vi "ActionVIOnLoad.vi"(8 "error in":errorcluster, 11 "Device Item Ref in":T1 format="%.0x") -> (0 "error out":errorcluster, 3 "Device Item Ref out":T1 format="%.0x")   [LabVIEW 2020, in "AIM MIL-STD-1553 System Explorer.lvlib" / "Implementation.lvlib"]
uses:
  Implementation.lvlib
  <vilib>/NI VeriStand/Custom Device API/Custom Device API.lvlib
  NationalInstruments.VeriStand.SystemDefinitionAPI
  Scripting/AIM MIL-STD-1553 Scripting.lvlib
  <vilib>/NI VeriStand/Custom Device API/Custom Device Item Ref.ctl
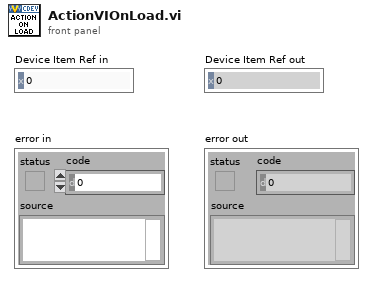
[diagram p1: front panel]
types:
  T1 = typedef "Custom Device API.lvlib/Custom Device Item Ref.ctl" = u64
  T2 = typedef "Custom Device API.lvlib/Custom Device Item Info.ctl" = cluster{"Name":string, "Is Channel":bool, "GUID":string, "Is Waveform":bool}
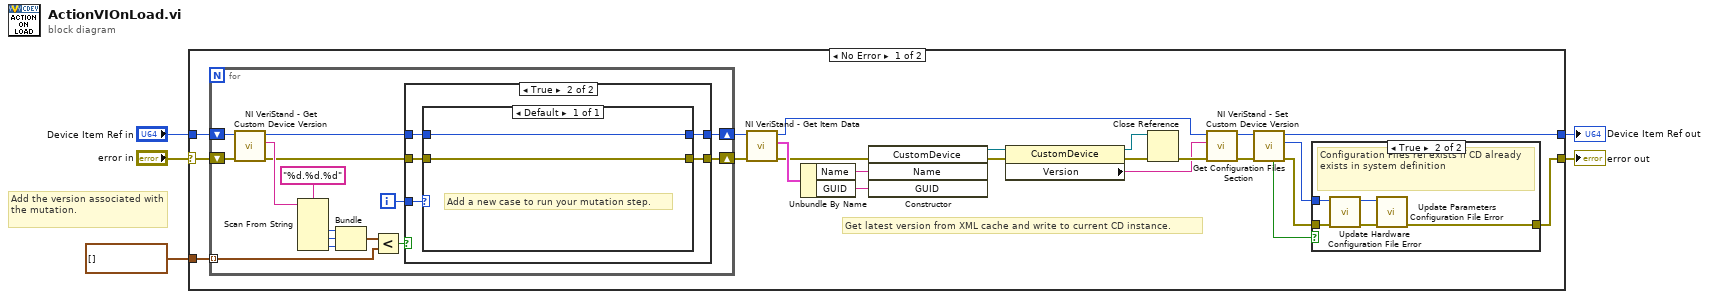
[diagram p0: block diagram]
diagram:
  # "Add the version associated with the mutation."
  n1 = case shown="No Error" "error in" {
    selector: "error in" -> [w28 w60]
    tunnel: [w8 w60] -> w3
    tunnel: "Device Item Ref in" -> [w27 w59]
    tunnel: [w7 w59] -> w2
    tunnel: cluster{i32, i32, i32}[] [] -> [w26 _]
    frame No Error {
      # "Get latest version from XML cache and write to current CD instance."
      n2 = for {
        shift-right: [w40] -> w24
        shift-left: w28 -> [w45]
        shift-right: [w38] -> w25
        shift-left: w27 -> [w44]
        tunnel: w26 -> [w35] mode=indexing
        i -> [w37]
        n3 = call <vilib>:"NI VeriStand - Get Custom Device Version.vi"("error in (no error)"=w45, "Device Ref in"=w44) -> ("error out"=w41:errorcluster, "Value"=w43:string, "Device Ref out"=w39:T1)  [unwired: 7 in]
        n4 = Scan From String(format string="%d.%d.%d", input string=w43) -> (output 1=w47:i32, output 2=w48:i32, output 3=w36:i32)  [unwired: 5 in, 3 out]
        n5 = Bundle(w47, w48, w36) -> (w49:cluster{i32, i32, i32})  [unwired: 1 in]
        n6 = Less?(x=w49, y=w35) -> (x < y?=w42:bool)
        n7 = case shown="True" w42 {
          tunnel: w41 -> [w51 w56]
          tunnel: [w51 w55] -> w40
          tunnel: w39 -> [w50 w52]
          tunnel: [w50 w53] -> w38
          tunnel: w37 -> [_ w54]
          frame False {
          }
          frame True {
            n8 = case shown="Default" w54 {
              tunnel: w56 -> [w58]
              tunnel: [w58] -> w55
              tunnel: [w57] -> w53
              tunnel: w52 -> [w57]
              frame Default {
                # "Add a new case to run your mutation step."
              }
            }
          }
        }
      }
      n9 = call <vilib>:"NI VeriStand - Get Item Data.vi"("error in (no error)"=w24, "Item Ref in"=w25) -> ("error out"=w20:errorcluster, "Item Info"=w23:T2, "Item Ref out"=w13:T1)  [unwired: 6 in, 1 out]
      n10 = Unbundle By Name(w23) -> ("Name"=w22:string, "GUID"=w21:string)
      n11 = constructor class="CustomDevice"(error in=w20, "Name"=w22, "GUID"=w21) -> (reference out=w19:refnum<k24>, error out=w18:errorcluster)  [unwired: 2 in, 3 out]
      n12 = property class="CustomDevice"(reference=w19, error in=w18) -> (reference out=w16:refnum<k24>, error out=w17:errorcluster, "Version"=w14:string)
      n13 = Close Reference(reference=w16, error in (no error)=w17) -> (error out=w15:errorcluster)
      n14 = call <vilib>:"NI VeriStand - Set Custom Device Version.vi"("error in (no error)"=w15, "Value"=w14, "Device Ref in"=w13) -> ("error out"=w11:errorcluster, "Device Ref out"=w12:T1)  [unwired: 7 in]
      n15 = call "Get Configuration Files Section.vi"("error in"=w11, "custom device in"=w12) -> ("error out"=w10:errorcluster, "configuration files section"=w9:T1, "custom device out"=w7:T1, "found"=w6:bool)  [unwired: 6 in]
      n16 = case shown="True" w6 {
        tunnel: w10 -> [w29 w34]
        tunnel: w9 -> [_ w33]
        tunnel: [w29 w30] -> w8
        frame False {
          # "expected when a new CD created"
        }
        frame True {
          # "Configuration Files ref exists if CD already exists in system definition"
          n17 = call "Update Hardware Configuration File Error.vi"("error in"=w34, "configuration files ref in"=w33) -> ("error out"=w31:errorcluster, "configuration files ref out"=w32:T1)  [unwired: 8 in]
          n18 = call "Update Parameters Configuration File Error.vi"("error in"=w31, "configuration files ref in"=w32) -> ("error out"=w30:errorcluster)  [unwired: 8 in, 1 out]
        }
      }
    }
    frame Error {
    }
  }
  "error out" <- w3
  "Device Item Ref out" <- w2
